vi "Add Text Token.vi"(8 "Error In":errorcluster, 11 "Lexer In":refnum<class "Lexer.lvclass">) -> (0 "Error Out":errorcluster, 3 "Lexer Out":refnum<class "Lexer.lvclass">)   [LabVIEW 2018, in "Toolkit.lvlib" / "Lexer.lvclass"]
uses:
  Lexer.lvclass
  Lexer.lvclass/Lexer.ctl
  Tokens/Text/Text.lvclass
  D:/Users/cfield/Code/Field R&D Services/Labstache/src/Toolkit/Low-Level/Tokens/Token/Token.lvclass
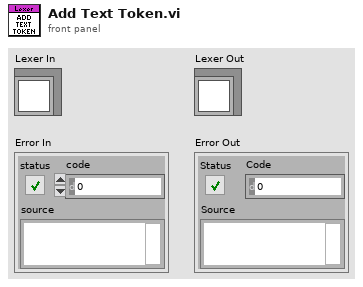
[diagram p1: front panel]
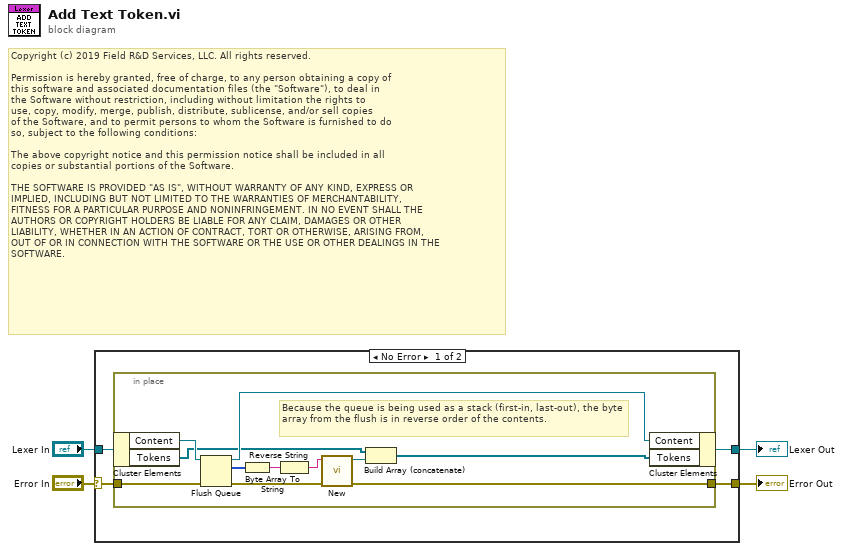
[diagram p0: block diagram]
diagram:
  # "Copyright (c) 2019 Field R&D Services, LLC. All rights reserved.\n\nPermission is hereby granted, free of charge, to any person obtaining a copy of\nthis software and associated documentation files (the \"Software\"), to deal in\nthe Software without restriction, including without limitation the rights to\nuse, copy, modify, merge, publish, distribute, sublicense, and/or sell copies\nof the Software, and to permit persons to whom the Software is furnished to do\nso, subject to the following conditions:\n\nThe above copyright notice and this permission notice shall be included in all\ncopies or substantial portions of the Software.\n\nTHE SOFTWARE IS PROVIDED \"AS IS\", WITHOUT WARRANTY OF ANY KIND, EXPRESS OR\nIMPLIED, INCLUDING BUT NOT LIMITED TO THE WARRANTIES OF MERCHANTABILITY,\nFITNESS FOR A PARTICULAR PURPOSE AND NONINFRINGEMENT. IN NO EVENT SHALL THE\nAUTHORS OR COPYRIGHT HOLDERS BE LIABLE FOR ANY CLAIM, DAMAGES OR OTHER\nLIABILITY, WHETHER IN AN ACTION OF CONTRACT, TORT OR OTHERWISE, ARISING FROM,\nOUT OF OR IN CONNECTION WITH THE SOFTWARE OR THE USE OR OTHER DEALINGS IN THE\nSOFTWARE."
  n1 = case shown="No Error" "Error In" {
    selector: "Error In" -> [w6 w20]
    tunnel: [w5 w20] -> w4
    tunnel: [w8 w21] -> w3
    tunnel: "Lexer In" -> [w7 w21]
    frame No Error {
      n2 = in-place {
        in-place-border: w6 -> [w13]
        in-place-border: [w9] -> w5
        # "Because the queue is being used as a stack (first-in, last-out), the byte array from the flush is in reverse order of the contents."
        n3 = in-place-cluster #1(w7) -> ("Content"=w19:refnum<queue>, "Tokens"=w16:refnum<class "Token.lvclass">[])
        n4 = Flush Queue(queue=w19, error in (no error)=w13) -> (queue out=w18:refnum<queue>, remaining elements=w17:u8[], error out=w10:errorcluster)
        n5 = Byte Array To String(unsigned byte array=w17) -> (string=w12:string)
        n6 = Reverse String(1:w12) -> (0:w11:string)
        n7 = call "New.vi"("Error In"=w10, "Content"=w11) -> ("Error Out"=w9:errorcluster, "Text"=w15:refnum<class "Text.lvclass">)  [unwired: 8 in]
        n8 = Build Array (concatenate)(w16, w15) -> (w14:refnum<class "Token.lvclass">[])
        n9 = in-place-cluster #1("Content"=w18, "Tokens"=w14) -> (w8:refnum<class "Lexer.lvclass">)
      }
    }
    frame Error {
    }
  }
  "Error Out" <- w4
  "Lexer Out" <- w3
